vi "Flush Queues.vi"(8 "error in":errorcluster, 10 "RTD":T2, 11 "MFB":T1) -> (0 "error out":errorcluster)   [LabVIEW 2022 SP3]
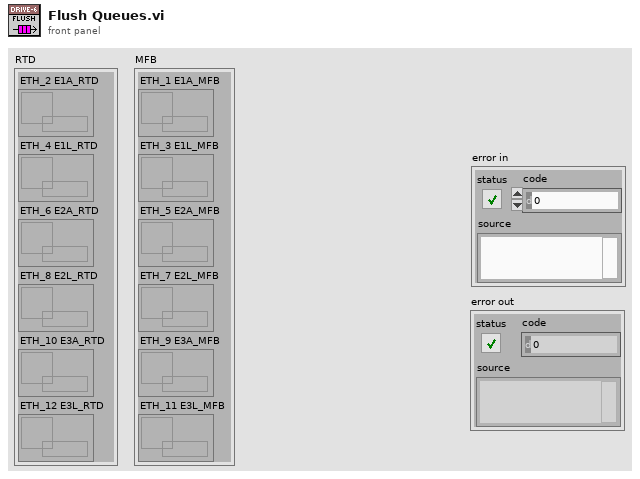
[diagram p1: front panel]
types:
  T1 = cluster{"ETH_1 E1A_MFB":refnum<queue>, "ETH_3 E1L_MFB":refnum<queue>, "ETH_5 E2A_MFB":refnum<queue>, "ETH_7 E2L_MFB":refnum<queue>, "ETH_9 E3A_MFB":refnum<queue>, "ETH_11 E3L_MFB":refnum<queue>}
  T2 = cluster{"ETH_2 E1A_RTD ":refnum<queue>, "ETH_4 E1L_RTD ":refnum<queue>, "ETH_6 E2A_RTD ":refnum<queue>, "ETH_8 E2L_RTD ":refnum<queue>, "ETH_10 E3A_RTD ":refnum<queue>, "ETH_12 E3L_RTD ":refnum<queue>}
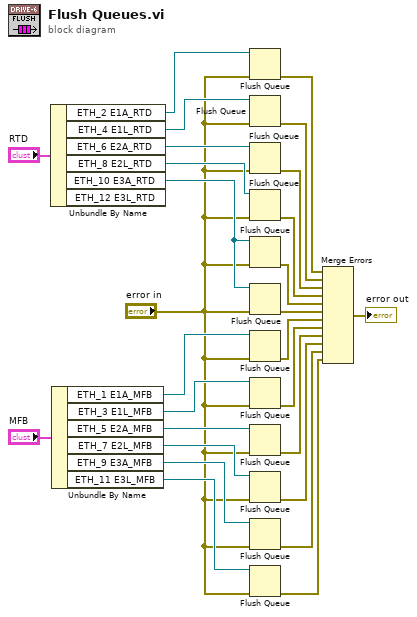
[diagram p0: block diagram]
diagram:
  n1 = Unbundle By Name("RTD") -> ("ETH_2 E1A_RTD"=w19:refnum<queue>, "ETH_4 E1L_RTD"=w18:refnum<queue>, "ETH_6 E2A_RTD"=w17:refnum<queue>, "ETH_8 E2L_RTD"=w16:refnum<queue>, "ETH_10 E3A_RTD"=w15:refnum<queue>)  [unwired: 1 out]
  n2 = Unbundle By Name("MFB") -> ("ETH_1 E1A_MFB"=w26:refnum<queue>, "ETH_3 E1L_MFB"=w25:refnum<queue>, "ETH_5 E2A_MFB"=w24:refnum<queue>, "ETH_7 E2L_MFB"=w23:refnum<queue>, "ETH_9 E3A_MFB"=w22:refnum<queue>, "ETH_11 E3L_MFB"=w21:refnum<queue>)
  n3 = Flush Queue(queue=w19, error in (no error)="error in") -> (error out=w13:errorcluster)  [unwired: 2 out]
  n4 = Flush Queue(queue=w18, error in (no error)="error in") -> (error out=w12:errorcluster)  [unwired: 2 out]
  n5 = Flush Queue(queue=w17, error in (no error)="error in") -> (error out=w11:errorcluster)  [unwired: 2 out]
  n6 = Flush Queue(queue=w16, error in (no error)="error in") -> (error out=w10:errorcluster)  [unwired: 2 out]
  n7 = Flush Queue(queue=w15, error in (no error)="error in") -> (error out=w9:errorcluster)  [unwired: 2 out]
  n8 = Flush Queue(queue=w15, error in (no error)="error in") -> (error out=w8:errorcluster)  [unwired: 2 out]
  n9 = Flush Queue(queue=w26, error in (no error)="error in") -> (error out=w7:errorcluster)  [unwired: 2 out]
  n10 = Flush Queue(queue=w25, error in (no error)="error in") -> (error out=w6:errorcluster)  [unwired: 2 out]
  n11 = Flush Queue(queue=w24, error in (no error)="error in") -> (error out=w5:errorcluster)  [unwired: 2 out]
  n12 = Flush Queue(queue=w23, error in (no error)="error in") -> (error out=w4:errorcluster)  [unwired: 2 out]
  n13 = Flush Queue(queue=w22, error in (no error)="error in") -> (error out=w3:errorcluster)  [unwired: 2 out]
  n14 = Flush Queue(queue=w21, error in (no error)="error in") -> (error out=w2:errorcluster)  [unwired: 2 out]
  n15 = Merge Errors(w13, w12, w11, w10, w9, w8, w7, w6, w5, w4, w3, w2) -> (→"error out":errorcluster)
